vi "Get 4-Rayleigh Parameters(SubVI).vi"(6 "Flow Peak Amp.":dbl, 8 "T_Flow Start (s)":dbl, 9 "T_Flow Peak (s)":dbl, 10 "T_Ejection period (s)":dbl, 11 "Pressure (mmHg)":waveform(dbl)) -> (3 "Optimised Parameter":dbl[](array[numeric]))   [LabVIEW 2017]
uses:
  72fe1329-4430-4fd7-86c8-dfab2f7b2d2e.vi
  5c84d562-1cd3-438d-9587-7d7d9e0fcbf7.vi
panel:
  out "sorted 2D array":dbl[][](array[numeric])
  out "x-1":i32
  out "sorted array of params":dbl[][](array[numeric])
  out "Error Checks":dbl[][](array[numeric])
  out "Parameters":dbl[][](array[numeric])
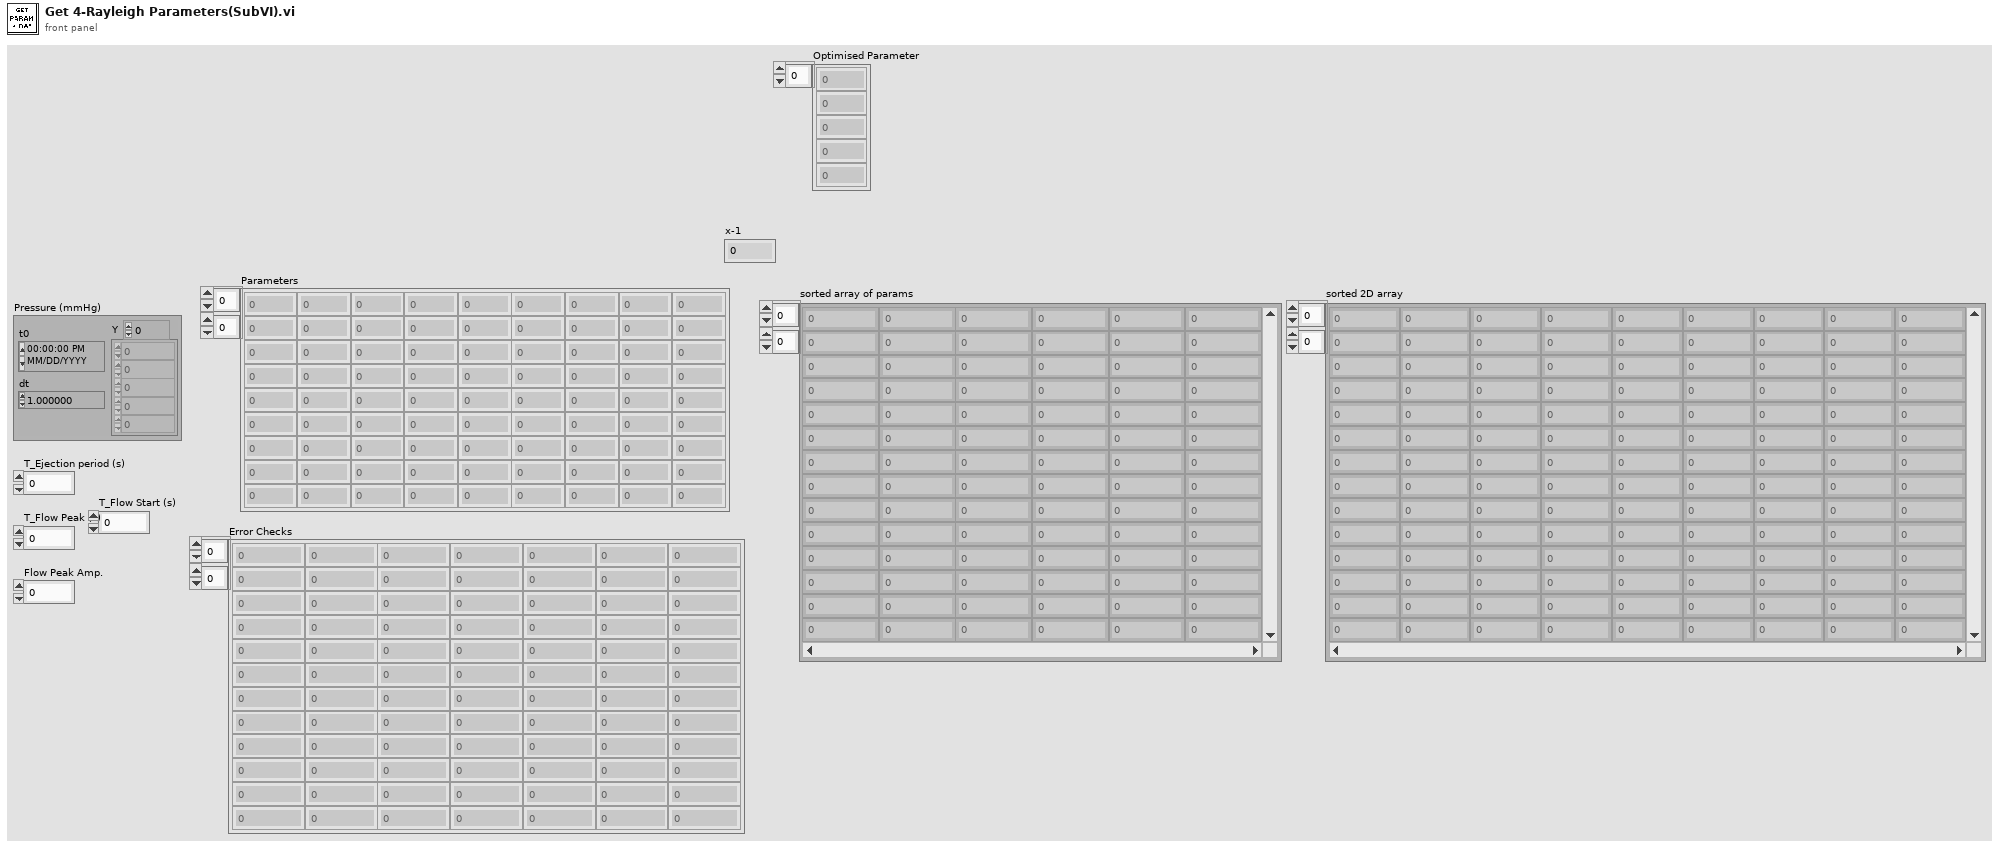
[diagram p1: front panel]
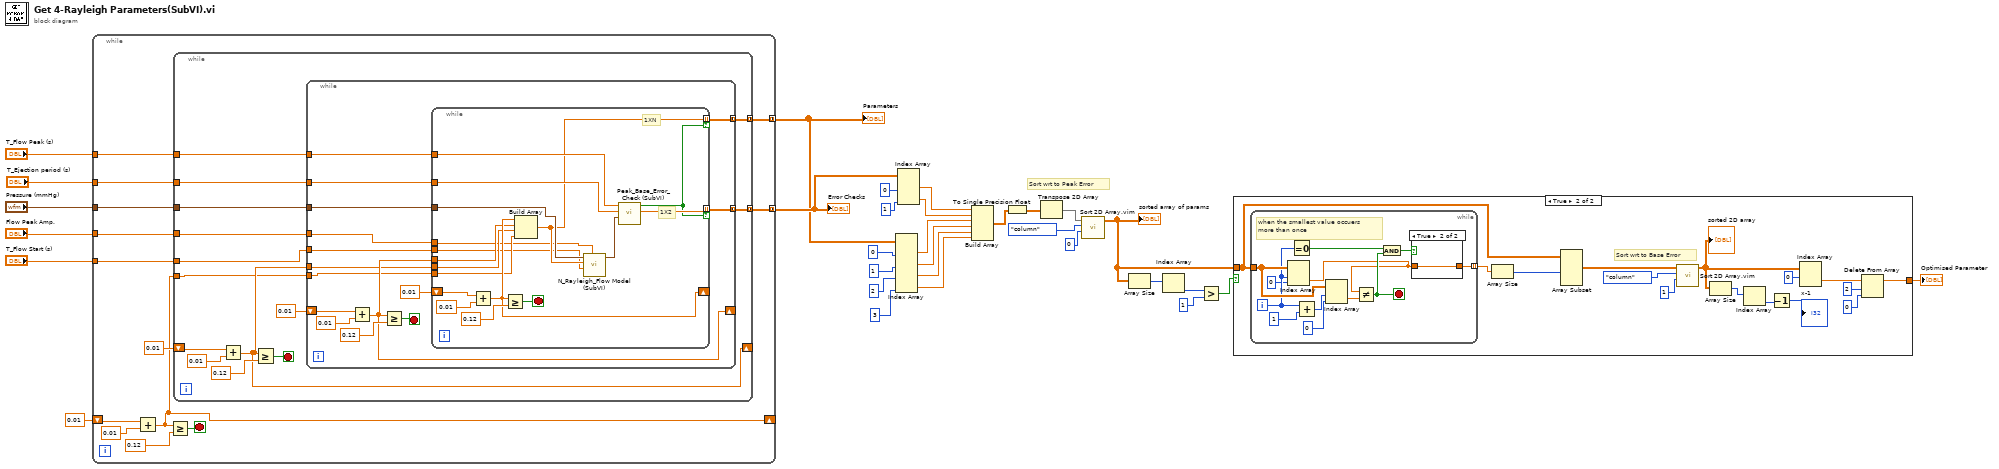
[diagram p0: block diagram]
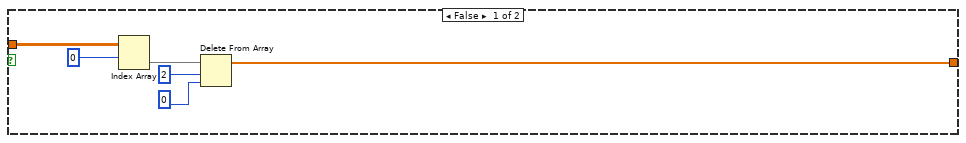
[diagram p2: hidden frame]
diagram:
  # "Sort wrt to Peak Error"
  n1 = while {
    tunnel: "Pressure (mmHg)" -> [w44]
    tunnel: "Flow Peak Amp." -> [w43]
    tunnel: "T_Ejection period (s)" -> [w42]
    tunnel: "T_Flow Peak (s)" -> [w41]
    tunnel: [w40] -> w21 mode=concatenating
    tunnel: [w39] -> w16 mode=concatenating
    tunnel: "T_Flow Start (s)" -> [w38]
    shift-right: [w32] -> _
    shift-left: 0.01 ("start") -> [w35]
    stop <- w33 stop-if-true
    n2 = Add(x=w35, y=0.01 ("start")) -> (x+y=w32:dbl)
    n3 = Greater Or Equal?(x=w32, y=0.12 ("start")) -> (x >= y?=w33:bool)
    n4 = while {
      tunnel: w44 -> [w58]
      tunnel: w43 -> [w57]
      tunnel: w42 -> [w55]
      tunnel: w41 -> [w54]
      tunnel: [w53] -> w40 mode=concatenating
      tunnel: [w52] -> w39 mode=concatenating
      tunnel: w38 -> [w51]
      shift-right: [w46] -> _
      shift-left: 0.01 ("start") -> [w48]
      tunnel: w32 -> [w45]
      stop <- w47 stop-if-true
      n5 = Add(x=w48, y=0.01 ("start")) -> (x+y=w46:dbl)
      n6 = Greater Or Equal?(x=w46, y=0.12 ("start")) -> (x >= y?=w47:bool)
      n7 = while {
        tunnel: w58 -> [w73]
        tunnel: w57 -> [w72]
        shift-right: [w67] -> _
        shift-left: 0.01 ("start") -> [w70]
        tunnel: w55 -> [w65]
        tunnel: w54 -> [w64]
        tunnel: [w63] -> w52 mode=concatenating
        tunnel: [w62] -> w53 mode=concatenating
        tunnel: w51 -> [w61]
        tunnel: w46 -> [w60]
        tunnel: w45 -> [w59]
        stop <- w68 stop-if-true
        n8 = Add(x=w70, y=0.01 ("start")) -> (x+y=w67:dbl)
        n9 = Greater Or Equal?(x=w67, y=0.12 ("start")) -> (x >= y?=w68:bool)
        n10 = while {
          tunnel: w73 -> [w78]
          tunnel: w72 -> [w75]
          tunnel: w67 -> [w81]
          shift-right: [w82] -> _
          shift-left: 0.01 ("start") -> [w88]
          tunnel: w65 -> [w86]
          tunnel: w64 -> [w85]
          tunnel: [w77] -> w63 mode=indexing if=w83
          tunnel: [w84] -> w62 mode=indexing if=w83
          tunnel: w61 -> [w76]
          tunnel: w60 -> [w80]
          tunnel: w59 -> [w79]
          stop <- w87 stop-if-true
          # "1X2"
          # "1XN"
          n11 = Add(x=w88, y=0.01 ("start")) -> (x+y=w82:dbl)
          n12 = Greater Or Equal?(x=w82, y=0.12 ("start")) -> (x >= y?=w87:bool)
          n13 = Build Array(w82, w81, w80, w79) -> (w77:dbl[])
          n14 = call "N_Rayleigh_Flow Model (SubVI).vi"("PSQ (ml/s)"=w75, "T_Flow Start"=w76, "Parameters (1XN)"=w77, "Pressure (mmHg)"=w78) -> ("n-Rayleigh Model Flow"=w74:waveform(dbl))  [unwired: 4 in, 1 out]
          n15 = call "Peak_Base_Error_Check (SubVI).vi"("Model Flow"=w74, "T_Ejection Period (s)"=w86, "T_Flow Peak (s)"=w85) -> ("Error"=w84:dbl[], "Logic"=w83:bool)  [unwired: 5 in, 2 out]
        }
      }
    }
  }
  "Parameters" <- w16
  "Error Checks" <- w21
  n16 = Index Array(array=w16, index (col) #1=0 ("disabled index (col)"), index (col) #2=1 ("index (col)"), index (col) #3=2 ("index (col)"), index (col) #4=3 ("index (col)")) -> (element #1=w18:dbl[], element #2=w17:dbl[], element #3=w4:dbl[], element #4=w1:dbl[])  [unwired: 4 in]
  n17 = Index Array(array=w21, index (col) #1=0 ("disabled index (col)"), index (col) #2=1 ("index (col)")) -> (element #1=w20:dbl[], element #2=w19:dbl[])  [unwired: 2 in]
  n18 = Build Array(w20, w19, w18, w17, w4, w1) -> (w7:dbl[][])
  n19 = To Single Precision Float(number=w7) -> (single precision float=w8:sgl[][])
  n20 = Transpose 2D Array(2D array=w8) -> (transposed array=w15:sgl[][])
  n21 = call "Sort 2D Array.vim"("index"=0, "dimension to index (column)"=enum16{"column", "row"}."column", "2D array"=w15) -> ("sorted 2D array"=w9:sgl[][])  [unwired: 7 in, 1 out]
  "sorted array of params" <- w9
  n22 = Array Size(array=w9) -> (size(s)=w13:i32[])
  n23 = Index Array(array=w13) -> (element=w12:i32)  [unwired: 1 in]
  n24 = Greater?(x=w12, y=1) -> (0:w11:bool)
  n25 = case shown="True" w11 {
    tunnel: w9 -> [w96 w100]
    tunnel: [w91 w99] -> w10
    frame False {
      n26 = Index Array(array=w96, index (row)=0) -> (element=w94:sgl[])  [unwired: 1 in]
      n27 = Delete From Array(array=w94, length=2, index=0) -> (array with subset deleted=w91:sgl[])  [unwired: 1 out]
    }
    frame True {
      # "Sort wrt to Base Error"
      n28 = while {
        tunnel: w100 -> [w121]
        tunnel: [w118] -> w101 mode=indexing
        i -> [w120]
        stop <- w114 stop-if-true
        # "when the smallest value occuers \nmore than once"
        n29 = Index Array(array=w121, index (row)=w120, index (col)=0 ("disabled index (col)")) -> (element=w113:sgl)
        n30 = Equal To 0?(x=w120) -> (x = 0?=w119:bool)
        n31 = Add(x=w120, y=1) -> (x+y=w122:i32)
        n32 = Index Array(array=w121, index (row)=w122, index (col)=0 ("disabled index (col)")) -> (element=w112:sgl)
        n33 = Not Equal?(x=w113, y=w112) -> (x != y?=w114:bool)
        n34 = And(x=w119, y=w114) -> (x .and. y?=w115:bool)
        n35 = case shown="True" w115 {
          tunnel: w113 -> [w124 w125]
          tunnel: [w124 w125] -> w118
          frame False {
          }
          frame True {
          }
        }
      }
      n36 = Array Size(array=w101) -> (size(s)=w98:i32)
      n37 = Array Subset(array=w100, length (row)=w98) -> (w106:sgl[][])  [unwired: 3 in]
      n38 = call "Sort 2D Array.vim"("index"=1, "dimension to index (column)"=enum16{"column", "row"}."column", "2D array"=w106) -> ("sorted 2D array"=w107:sgl[][])  [unwired: 7 in, 1 out]
      "sorted 2D array" <- w107
      n39 = Array Size(array=w107) -> (size(s)=w108:i32[])
      n40 = Index Array(array=w108) -> (element=w109:i32)  [unwired: 1 in]
      n41 = Decrement(x=w109) -> (x-1=→"x-1":i32)
      n42 = Index Array(array=w107, index (row)=0) -> (element=w111:sgl[])  [unwired: 1 in]
      n43 = Delete From Array(array=w111, length=2, index=0) -> (array with subset deleted=w99:sgl[])  [unwired: 1 out]
    }
  }
  "Optimised Parameter" <- w10
